vi "Menue Tags auslesen.vi"(8 "error in (no error)":errorcluster caption="Fehler (Eingang, kein Fehler)", 11 "Menü Referenz":refnum<k9>) -> (0 "error out":errorcluster caption="Fehler (Ausgang)", 2 "Menu Tags":string[](array[string]), 3 "Menü Referenz out":refnum<k9>)   [LabVIEW 2020, in "Sprachverwaltung.lvlib"]
doc: "Liest die Runtime Menu und Submenu Tags aus und ersetzt die manuelle StringArray Liste.\nGefunden als deaktivierten Baustein im alten Sprachaschmodder ... stimmt aber mit vom NI Support empfohlenen Baustein überein.\n\nRIW - 31.08.2018"
uses:
  Sprachverwaltung.lvlib
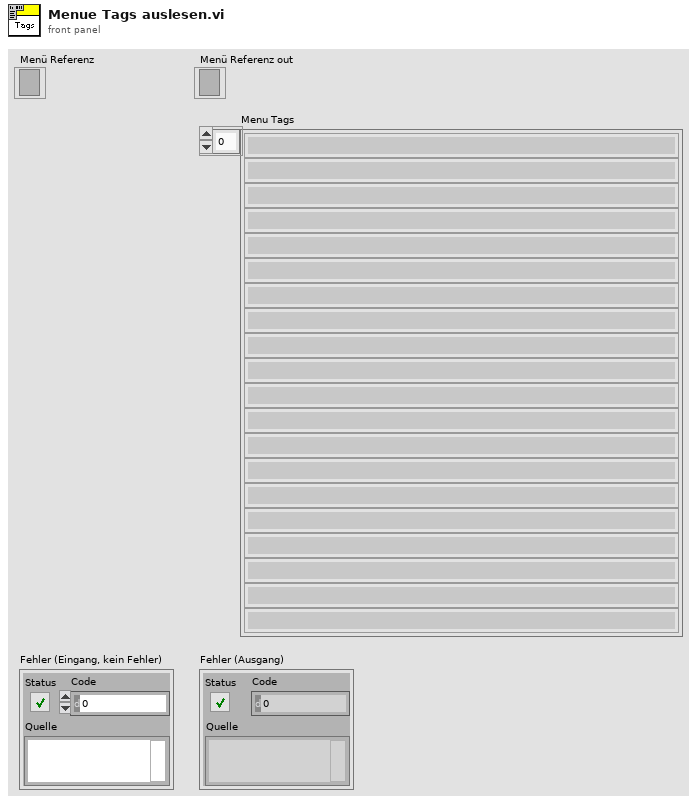
[diagram p1: front panel]
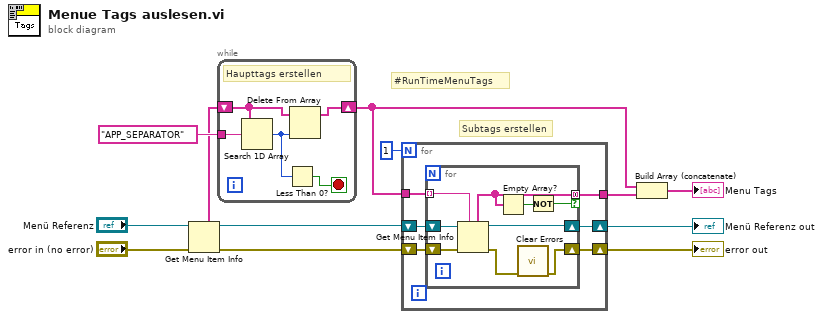
[diagram p0: block diagram]
diagram:
  # "#RunTimeMenuTags"
  # "Subtags erstellen"
  n1 = Get Menu Item Info(8:"error in (no error)", 11:"Menü Referenz") -> (0:w3:errorcluster, 3:w9:refnum<k9>, 5:w7:string[])  [unwired: 1 in, 4 out]
  n2 = while {
    tunnel: "APP_SEPARATOR" -> [w17]
    shift-right: [w15] -> w11
    shift-left: w7 -> [w16]
    stop <- w14 stop-if-true
    # "Haupttags erstellen"
    n3 = Search 1D Array(1D array=w16, element=w17) -> (index of element=w13:i32)  [unwired: 1 in]
    n4 = Less Than 0?(x=w13) -> (x < 0?=w14:bool)
    n5 = Delete From Array(array=w16, index=w13) -> (array with subset deleted=w15:string[])  [unwired: 1 in, 1 out]
  }
  n6 = for {
    N: 1 -> [_]
    tunnel: w11 -> [w23]
    tunnel: [w21] -> w12
    shift-right: [w20] -> w2
    shift-left: w3 -> [w19]
    shift-right: [w18] -> w1
    shift-left: w9 -> [w22]
    n7 = for {
      tunnel: w23 -> [w32] mode=indexing
      tunnel: [w30] -> w21 mode=concatenating if=w28
      shift-right: [w26] -> w20
      shift-left: w19 -> [w25]
      shift-right: [w24] -> w18
      shift-left: w22 -> [w31]
      n8 = Get Menu Item Info(7:w32, 8:w25, 11:w31) -> (0:w27:errorcluster, 3:w24:refnum<k9>, 5:w30:string[])  [unwired: 4 out]
      n9 = Empty Array?(array=w30) -> (empty?=w29:bool)
      n10 = call <vilib>:"Clear Errors.vi"("error in (no error)"=w27) -> ("error out"=w26:errorcluster)  [unwired: 5 in, 1 out]
      n11 = Not(x=w29) -> (.not. x?=w28:bool)
    }
  }
  "error out" <- w2
  "Menü Referenz out" <- w1
  n12 = Build Array (concatenate)(w11, w12) -> (→"Menu Tags":string[])
